vi "Center Quadrant.vi"(1 "Array In":u16[][](array[numeric])) -> (0 "Center Quad":u16[][](array[numeric]))   [LabVIEW 2023]
panel:
  out "size(s)":i32[](array[numeric])
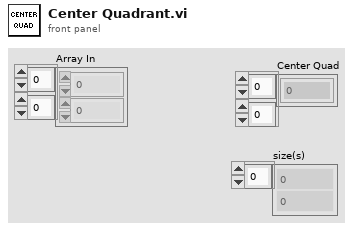
[diagram p1: front panel]
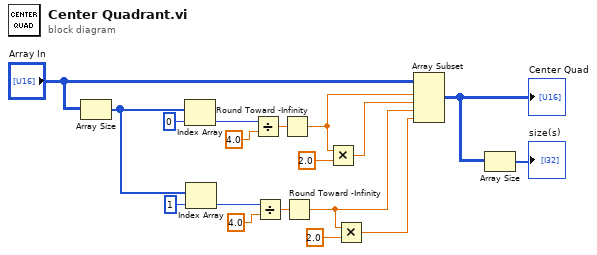
[diagram p0: block diagram]
diagram:
  n1 = Array Size(array="Array In") -> (size(s)=w14:i32[])
  n2 = Index Array(array=w14, index=0) -> (element=w15:i32)
  n3 = Index Array(array=w14, index=1) -> (element=w9:i32)
  n4 = Divide(x=w15, y=4.0) -> (x/y=w17:dbl)
  n5 = Divide(x=w9, y=4.0) -> (x/y=w10:dbl)
  n6 = Round Toward -Infinity(1:w17) -> (0:w7:dbl)
  n7 = Round Toward -Infinity(1:w10) -> (0:w5:dbl)
  n8 = Multiply(x=w7, y=2.0) -> (x*y=w6:dbl)
  n9 = Multiply(x=w5, y=2.0) -> (x*y=w4:dbl)
  n10 = Array Subset(array="Array In", index (row)=w7, length (row)=w6, index (col)=w5, length (col)=w4) -> (w3:u16[][])
  "Center Quad" <- w3
  n11 = Array Size(array=w3) -> (size(s)=→"size(s)":i32[])
